vi "Calibrate.vi"(9 "Voltages":sgl[](array[numeric]), 11 "CalCurrent":sgl) -> (0 "Done":bool, 3 "ProgressMsg":string)   [LabVIEW 2025]
uses:
  Globals.vi
  <vilib>/Analysis/NI_AALBase.lvlib
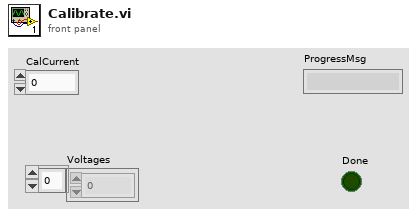
[diagram p1: front panel]
types:
  T1 = typedef "Mode.ctl" = enum16{"R1 Only", "Parallel", "Serial"}
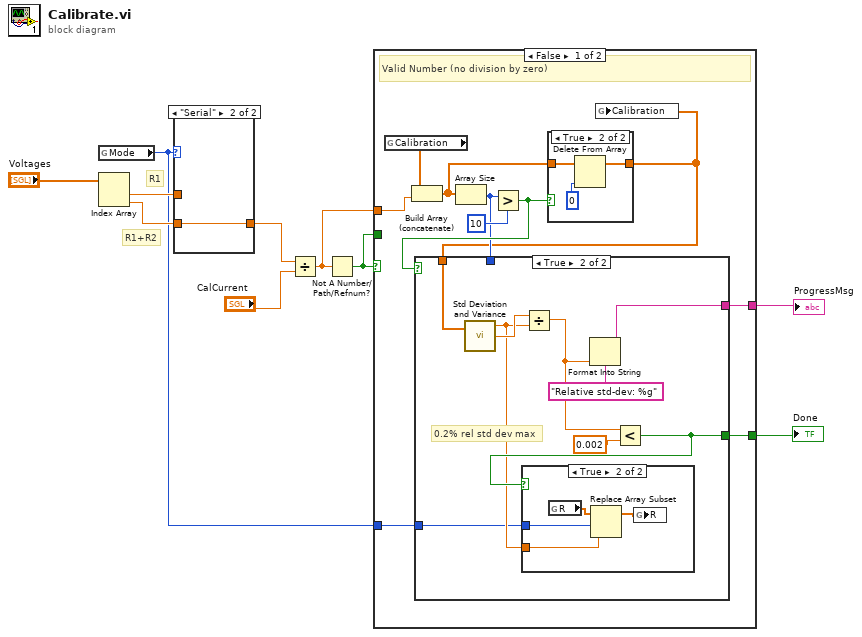
[diagram p0: block diagram]
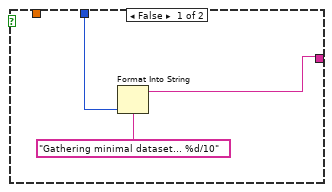
[diagram p2: hidden frame]
diagram:
  # "R1+R2"
  # "R1"
  n1 = global read "Globals.vi" "Mode"() -> (w1:T1)
  n2 = Index Array(array="Voltages") -> (element #1=w9:sgl, element #2=w8:sgl)  [unwired: 2 in]
  n3 = case shown="\"Serial\"" w1 {
    tunnel: [w11 w12] -> w7
    tunnel: w9 -> [w11 _]
    tunnel: w8 -> [_ w12]
    frame Default {
    }
    frame "Serial" {
    }
  }
  n4 = Divide(x=w7, y="CalCurrent") -> (x/y=w4:sgl)
  n5 = Not A Number/Path/Refnum?(number/path/refnum=w4) -> (NaN/Path/Refnum?=w5:bool)
  n6 = case shown="False" w5 {
    tunnel: w5 -> [_ _]
    tunnel: w4 -> [w21 _]
    tunnel: [w16 _] -> w3
    tunnel: [w14 _] -> w2
    tunnel: w1 -> [w13 _]
    frame False {
      # "Valid Number (no division by zero)"
      n7 = global read "Globals.vi" "Calibration"() -> (w22:sgl[])
      n8 = Build Array (concatenate)(w22, w21) -> (w19:sgl[])
      n9 = Array Size(array=w19) -> (size(s)=w17:i32)
      n10 = Greater?(x=w17, y=10) -> (0:w18:bool)
      n11 = case shown="True" w18 {
        tunnel: w19 -> [w39 w42]
        tunnel: [w39 w40] -> w15
        frame False {
        }
        frame True {
          n12 = Delete From Array(array=w42, index=0) -> (array with subset deleted=w40:sgl[])  [unwired: 1 in, 1 out]
        }
      }
      n13 = case shown="True" w18 {
        tunnel: w17 -> [w25 _]
        tunnel: [w23 w31] -> w16
        tunnel: w15 -> [_ w34]
        tunnel: [_ w29] -> w14
        tunnel: w13 -> [_ w26]
        frame False {
          n14 = Format Into String(format string="Gathering minimal dataset... %d/10", w25) -> (resulting string=w23:string)  [unwired: 2 in, 1 out]
        }
        frame True {
          # "0.2% rel std dev max"
          n15 = call <vilib>:"Std Deviation and Variance.vi"("X"=w34) -> ("mean"=w27:dbl, "standard deviation"=w33:dbl)  [unwired: 1 in, 1 out]
          n16 = Divide(x=w33, y=w27) -> (x/y=w28:dbl)
          n17 = Format Into String(format string="Relative std-dev: %g", w28) -> (resulting string=w31:string)  [unwired: 2 in, 1 out]
          n18 = Less?(x=w28, y=0.002) -> (x < y?=w29:bool)
          n19 = case shown="True" w29 {
            tunnel: w27 -> [_ w35]
            tunnel: w26 -> [_ w36]
            frame False {
            }
            frame True {
              n20 = global read "Globals.vi" "R"() -> (w38:dbl[])
              n21 = Replace Array Subset(array=w38, new element=w35, index=w36) -> (w37:dbl[])
              n22 = global write "Globals.vi" "R"(w37) -> ()
            }
          }
        }
      }
      n23 = global write "Globals.vi" "Calibration"(w15) -> ()
    }
    frame True {
    }
  }
  "Done" <- w2
  "ProgressMsg" <- w3
